vi "_GlobalSettings.vi"(6 "Oper(Get)":bool, 8 "error in (no error)":errorcluster, 11 "Setting in":T1) -> (0 "error out":errorcluster, 3 "Setting out":T1)   [LabVIEW 2017, in "MDPtr.lvlib"]
uses:
  MDPtr.lvlib
  Def-GlobalSettings.ctl
  MDPtr TypeDef/MDPtr MallocMethod.ctl
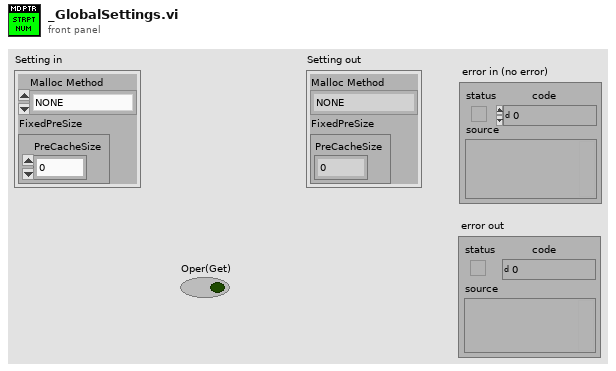
[diagram p1: front panel]
types:
  T1 = typedef "MDPtr.lvlib/Def-GlobalSettings.ctl" = cluster{"Malloc Method":T2, "FixedPreSize":cluster{"PreCacheSize":i32}}
  T2 = typedef "MDPtr.lvlib/MDPtr MallocMethod.ctl" = enum16{"NONE", "FIXED PRE-SIZE"}
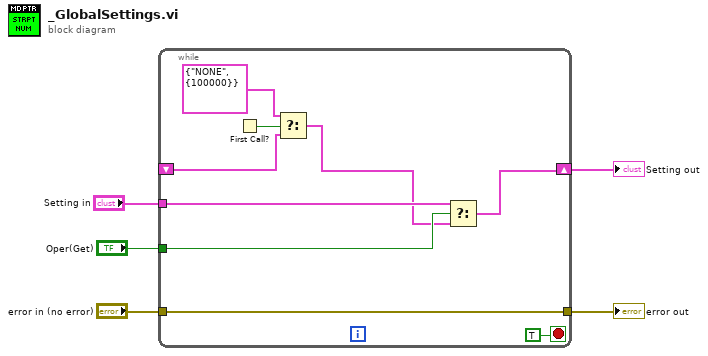
[diagram p0: block diagram]
diagram:
  n1 = while {
    tunnel: "Oper(Get)" -> [w11]
    shift-right: [w10] -> w4
    shift-left: _ -> [w7]
    tunnel: "error in (no error)" -> [w13]
    tunnel: [w13] -> w2
    tunnel: "Setting in" -> [w12]
    stop <- TRUE stop-if-true
    n2 = First Call?() -> (First Call?: T/F=w9:bool)
    n3 = Select(t=T1 {"Malloc Method"=enum."NONE", "FixedPreSize"={"PreCacheSize"=100000}} ("Cluster"), s=w9, f=w7) -> (s? t:f=w6:T1)
    n4 = Select(t=w12, s=w11, f=w6) -> (s? t:f=w10:T1)
  }
  "error out" <- w2
  "Setting out" <- w4
